vi "Rcv Cmd.vi"(8 "error in":errorcluster, 11 "CRDS in":refnum<class "CRDS.lvclass">) -> (0 "error out":errorcluster, 3 "CRDS out":refnum<class "CRDS.lvclass">)   [LabVIEW 2014, in "CRDS.lvclass"]
uses:
  CRDS.lvclass
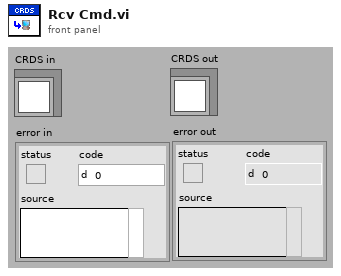
[diagram p1: front panel]
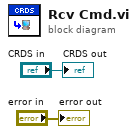
[diagram p0: block diagram]
diagram:
  "error out" <- "error in"
  "CRDS out" <- "CRDS in"
